vi "AlicatWrite8V0_modified.vi"(8 "error in (no error)":errorcluster, 9 "SetPoint (64000=FullScale)":i32=32000 min=0 max=64000 step=1, 10 "UnitID":string="A", 11 "VISA resource name":refnum<visa-resource-name>="COM1") -> (0 "error out":errorcluster={"status"=FALSE, "code"=0, "source"="VISA Read in ReadSerialBuffer.vi->AlicatSetPoint.vi->AlicatWrite8V2.vi"}, 1 "AlicatResponse":string="A +013.53 +023.20 +0000.0 +0000.0 0250.0     Air\r")   [LabVIEW 2011]
uses:
  <vilib>/Instr/_visa.llb/VISA Configure Serial Port (Instr).vi
panel:
  # "Read this response from the change the setpoint write.\nClears the Serial in buffer"
  # "Code 1073676294 is\nokay since we are only\nreading one byte till we\nget to the end of message\nbyte."
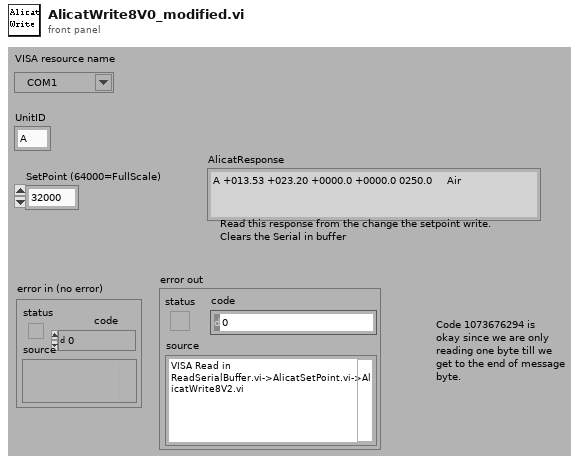
[diagram p1: front panel]
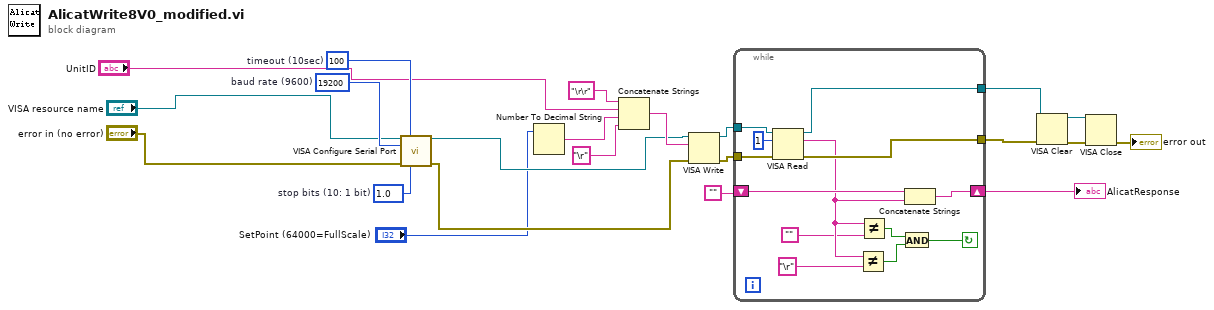
[diagram p0: block diagram]
diagram:
  w19 = u32 100  # timeout (10sec)
  w20 = u16 10 items=["1.0"=10, "1.5"=15, "2.0"=20]  # stop bits (10: 1 bit)
  w21 = u32 19200  # baud rate (9600)
  n1 = call-poly "VISA Configure Serial Port"("VISA resource name"="VISA resource name", "timeout (10sec)"=w19, "baud rate (9600)"=w21, "error in (no error)"="error in (no error)", "stop bits (10: 1 bit)"=w20) -> ("VISA resource name out"=w11:refnum<visa-resource-name>, "error out"=w10:errorcluster)  [unwired: 9 in]
  n2 = Number To Decimal String(number="SetPoint (64000=FullScale)") -> (decimal integer string=w14:string)  [unwired: 1 in]
  n3 = Concatenate Strings("\r\r" ("string"), "UnitID", w14, "\r" ("string")) -> (w16:string)
  n4 = VISA Write(VISA resource name=w11, write buffer=w16, error in (no error)=w10) -> (VISA resource name out=w2:refnum<visa-resource-name>, error out=w1:errorcluster)  [unwired: 1 out]
  n5 = while {
    tunnel: [w34] -> w7
    tunnel: [w33] -> w8
    shift-right: [w31] -> w3
    shift-left: "" -> [w30]
    tunnel: w2 -> [w24]
    tunnel: w1 -> [w23]
    stop <- w26 continue-if-true
    n6 = VISA Read(VISA resource name=w24, byte count=u32 1 ("byte count (0)"), error in (no error)=w23) -> (VISA resource name out=w33:refnum<visa-resource-name>, read buffer=w29:string, error out=w34:errorcluster)  [unwired: 1 out]
    n7 = Not Equal?(x=w29, y="\r") -> (x != y?=w27:bool)
    n8 = Not Equal?(x=w29, y="") -> (x != y?=w28:bool)
    n9 = And(x=w28, y=w27) -> (x .and. y?=w26:bool)
    n10 = Concatenate Strings(w30, w29) -> (w31:string)
  }
  "AlicatResponse" <- w3
  n11 = VISA Clear(VISA resource name=w8, error in (no error)=w7) -> (VISA resource name out=w5:refnum<visa-resource-name>, error out=w4:errorcluster)
  n12 = VISA Close(VISA resource name=w5, error in (no error)=w4) -> (error out=→"error out":errorcluster)
